vi "measure_volt.vi"() -> ()   [LabVIEW 2013]
uses:
  global_var.vi
panel:
  out "instrument ID":string
  out "voltage measures":string
  in  "stop":bool
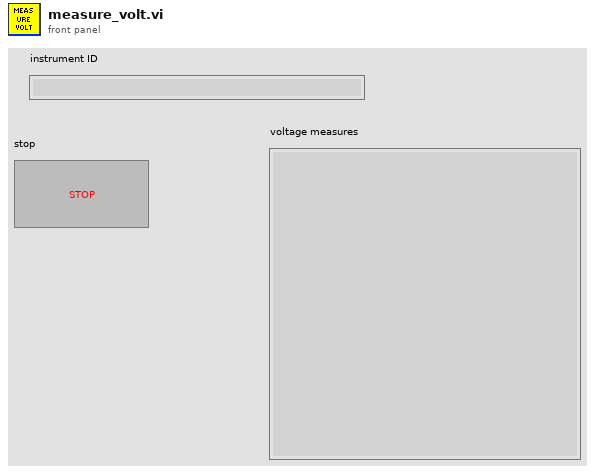
[diagram p1: front panel]
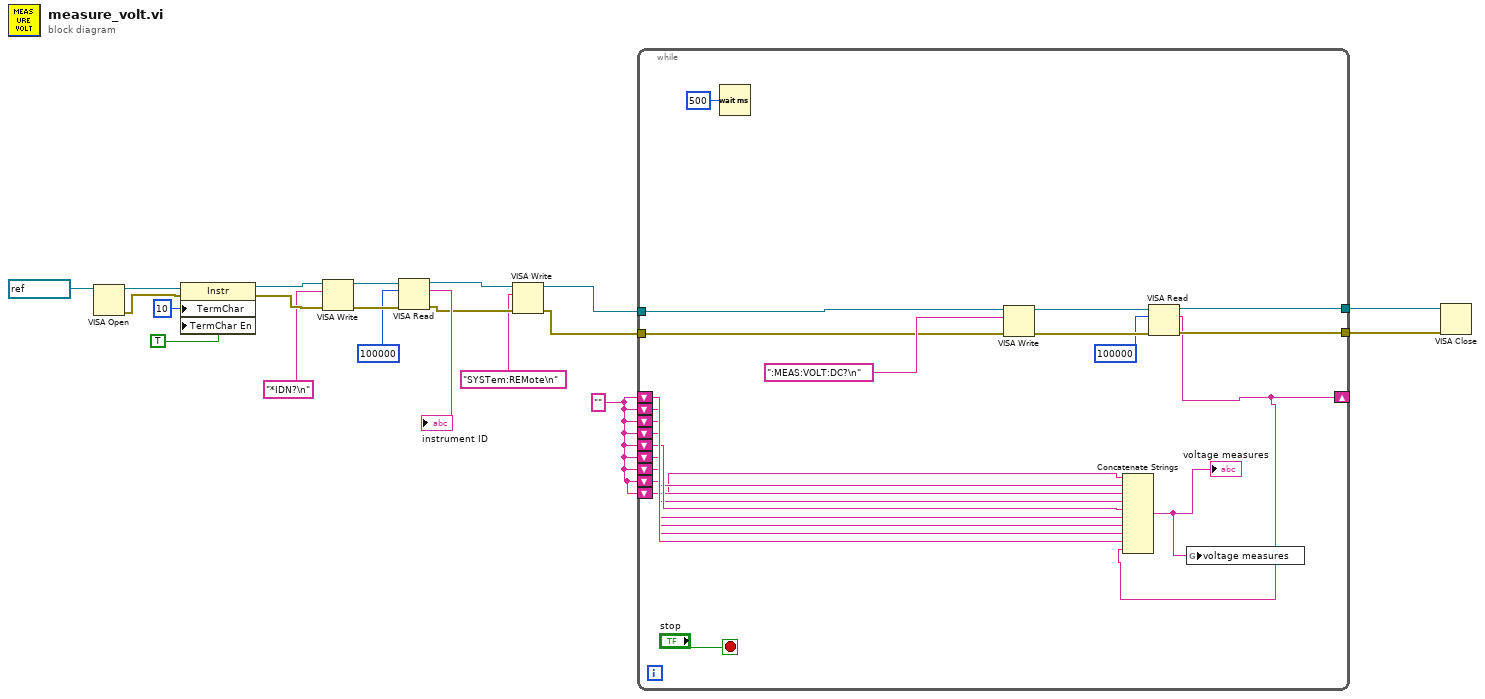
[diagram p0: block diagram]
diagram:
  w13 = ""
  n1 = VISA Open(VISA resource name=refnum<visa-resource-name> "COM3") -> (VISA resource name=w20:refnum<visa-resource-name>, error out=w17:errorcluster)  [unwired: 4 in]
  n2 = property class="Instr"(reference=w20, error in=w17, "TermChar"=u8 10 ("Message Based Settings:Termination Character"), "TermChar En"=TRUE ("Message Based Settings:Termination Character Enable")) -> (reference out=w12:refnum<visa-resource-name>, error out=w11:errorcluster)
  n3 = VISA Write(VISA resource name=w12, write buffer="*IDN?\n", error in (no error)=w11) -> (VISA resource name out=w9:refnum<visa-resource-name>, error out=w8:errorcluster)  [unwired: 1 out]
  n4 = VISA Read(VISA resource name=w9, byte count=u32 100000, error in (no error)=w8) -> (VISA resource name out=w5:refnum<visa-resource-name>, read buffer=→"instrument ID":string, error out=w4:errorcluster)  [unwired: 1 out]
  n5 = VISA Write(VISA resource name=w5, write buffer="SYSTem:REMote\n", error in (no error)=w4) -> (VISA resource name out=w2:refnum<visa-resource-name>, error out=w1:errorcluster)  [unwired: 1 out]
  n6 = while {
    tunnel: w2 -> [w40]
    tunnel: w1 -> [w38]
    tunnel: [w34] -> w16
    tunnel: [w33] -> w15
    shift-right: [w21] -> _
    shift-left: w13 -> [w31]
    shift-left: w13 -> [w30]
    shift-left: w13 -> [w29]
    shift-left: w13 -> [w28]
    shift-left: w13 -> [w27]
    shift-left: w13 -> [w26]
    shift-left: w13 -> [w25]
    shift-left: w13 -> [w24]
    shift-left: w13 -> [w23]
    stop <- "stop" stop-if-true
    n7 = Wait (ms)(milliseconds to wait=u32 500) -> ()  [unwired: 1 out]
    n8 = VISA Write(VISA resource name=w40, write buffer=":MEAS:VOLT:DC?\n", error in (no error)=w38) -> (VISA resource name out=w36:refnum<visa-resource-name>, error out=w37:errorcluster)  [unwired: 1 out]
    n9 = VISA Read(VISA resource name=w36, byte count=u32 100000, error in (no error)=w37) -> (VISA resource name out=w34:refnum<visa-resource-name>, read buffer=w21:string, error out=w33:errorcluster)  [unwired: 1 out]
    n10 = Concatenate Strings(w23, w24, w25, w26, w27, w28, w29, w30, w31, w21) -> (w22:string)
    "voltage measures" <- w22
    n11 = global write "global_var.vi" "voltage measures"(w22) -> ()
  }
  n12 = VISA Close(VISA resource name=w16, error in (no error)=w15) -> ()  [unwired: 1 out]
